vi "SHA-2-U64.vi"(7 "Type":T1, 8 "error in (no error)":errorcluster, 11 "Message":string="The quick brown fox jumps over the lazy dog") -> (0 "error out":errorcluster, 1 "ASCII Formatted hash":string, 3 "binary string hash":string caption="binary string (hex display)")   [LabVIEW 2012, in "Encryption.lvlib"]
doc: "Performs an SHA2 U64-bit.\n\n(c) Ton Plomp, 2011\nTHIS SOFTWARE IS PROVIDED AS IS, AND ANY WARRANTY IS REJECTED"
uses:
  Encryption.lvlib
  SHA-2_U64_types.ctl
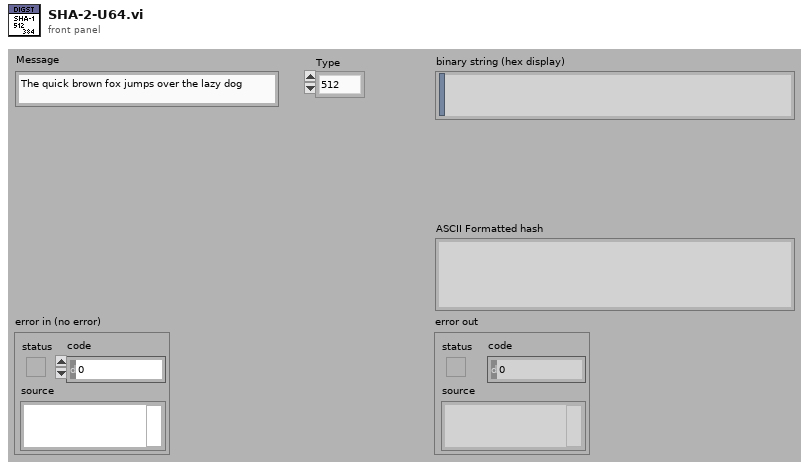
[diagram p1: front panel]
types:
  T1 = typedef "Encryption.lvlib/SHA-2_U64_types.ctl" = enum16{"512", "384"}
  T2 = enum16{"big-endian, network order", "native, host order", "little-endian"}
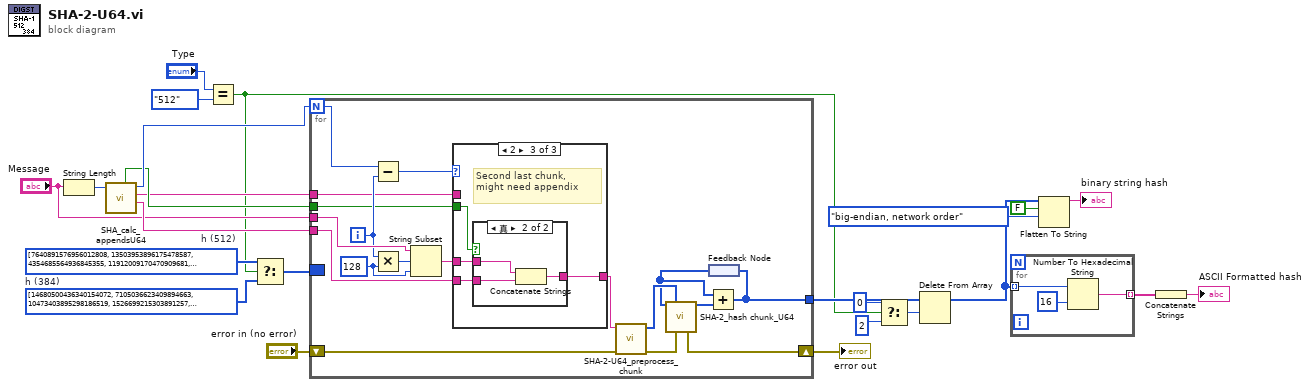
[diagram p0: block diagram]
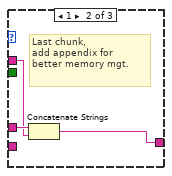
[diagram p3: hidden frame]
diagram:
  w6 = u64[] [14680500436340154072, 7105036623409894663, 10473403895298186519, 1526699215303891257, 7436329637833083697, 10282925794625328401, 15784041429090275239, 5167115440072839076]  # h (384)
  w10 = u64[] [7640891576956012808, 13503953896175478587, 4354685564936845355, 11912009170470909681, 5840696475078001361, 11170449401992604703, 2270897969802886507, 6620516959819538809]  # h (512)
  n1 = String Length(string="Message") -> (length=w1:i32)
  n2 = call "SHA_calc_appendsU64.vi"("String length"=w1) -> ("Second last chunk"=w18:string, "Last Chunk"=w19:string, "Number of chunks"=w21:i32, "Double appends"=w20:bool)  [unwired: 7 in]
  n3 = Equal?(x="Type", y=SHA-2_U64_types."512" ("Type")) -> (x = y?=w7:bool)
  n4 = Select(t=w10, s=w7, f=w6) -> (s? t:f=w9:u64[])
  n5 = for {
    N: w21 -> [w39]
    tunnel: "Message" -> [w42]
    tunnel: w19 -> [w35]
    tunnel: [w27] -> w8
    border: w9 -> [_]
    tunnel: w20 -> [w33]
    tunnel: w18 -> [w32]
    shift-right: [w31] -> w16
    shift-left: "error in (no error)" -> [w30]
    i -> [w38]
    w40 = 128 ("x")
    n6 = Subtract(x=w39, y=w38) -> (x-y=w36:i32)
    n7 = Multiply(x=w38, y=w40) -> (x*y=w41:i32)
    n8 = String Subset(string=w42, offset (0)=w41, length (rest)=w40) -> (substring=w37:string)
    n9 = case shown="2" w36 {
      tunnel: w37 -> [w43 w46 w50]
      tunnel: [w43 w44 w49] -> w25
      tunnel: w35 -> [_ w45 _]
      tunnel: w32 -> [_ _ w48]
      tunnel: w33 -> [_ _ w47]
      frame Default {
        # "Not last chunk"
      }
      frame 1 {
        # "Last chunk,\nadd appendix for\nbetter memory mgt."
        n10 = Concatenate Strings(w46, w45) -> (w44:string)
      }
      frame 2 {
        # "Second last chunk,\nmight need appendix"
        n11 = case shown="真" w47 {
          tunnel: w50 -> [w51 w54]
          tunnel: [w51 w53] -> w49
          tunnel: w48 -> [_ w52]
          frame False {
          }
          frame True {
            n12 = Concatenate Strings(w54, w52) -> (w53:string)
          }
        }
      }
    }
    n13 = call "SHA-2-U64_preprocess_chunk.vi"("error in (no error)"=w30, "Chunk in"=w25) -> ("error out"=w28:errorcluster, "Processed chunk out"=w29:u64[])  [unwired: 8 in]
    n14 = feedback #1() -> (w26:u64[])
    n15 = call "SHA-2_hash chunk_U64.vi"("h in"=w26, "Chunk"=w29, "error in (no error)"=w28) -> ("h out"=w34:u64[], "error out"=w31:errorcluster)  [unwired: 11 in]
    n16 = Add(x=w26, y=w34) -> (x+y=w27:u64[])
    n17 = feedback-in #1(w27) -> ()
  }
  "error out" <- w16
  n18 = Select(t=0, s=w7, f=2 ("length")) -> (s? t:f=w2:i32)
  n19 = Delete From Array(array=w8, length=w2) -> (array with subset deleted=w5:u64[])  [unwired: 1 in, 1 out]
  n20 = for {
    tunnel: w5 -> [w57] mode=indexing
    tunnel: [w55] -> w14 mode=indexing
    n21 = Number To Hexadecimal String(1:i16 16 ("width (-)"), 2:w57) -> (0:w55:string)
  }
  n22 = Flatten To String(anything=w5, prepend array or string size? (T)=FALSE, byte order (0:big-endian, network order)=T2."big-endian, network order") -> (data string=→"binary string hash":string)  [unwired: 1 in, 2 out]
  n23 = Concatenate Strings(w14) -> (→"ASCII Formatted hash":string)
